vi "Correlation_coefficient.vi"(0 "U":dbl[](array[numeric]) format="%.2f", 1 "W":dbl[](array[numeric]) format="%.2f") -> (17 "Correlation coefficient":dbl format="%.2f")   [LabVIEW 2010]
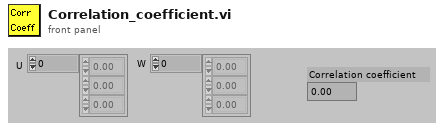
[diagram p1: front panel]
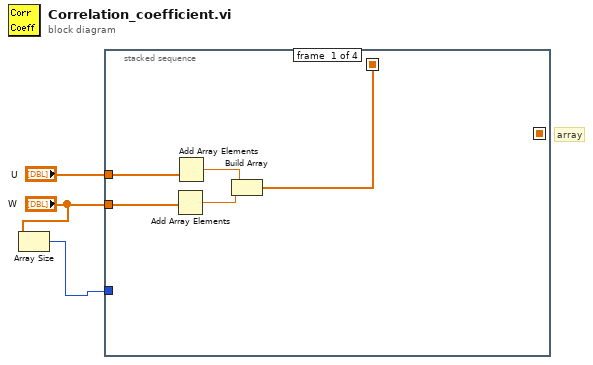
[diagram p0: block diagram]
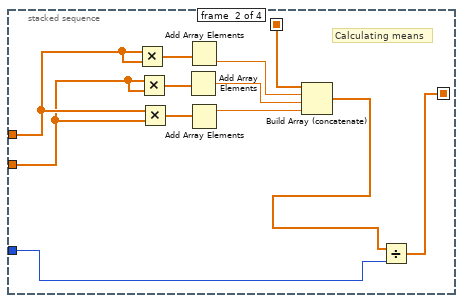
[diagram p2: hidden frame]
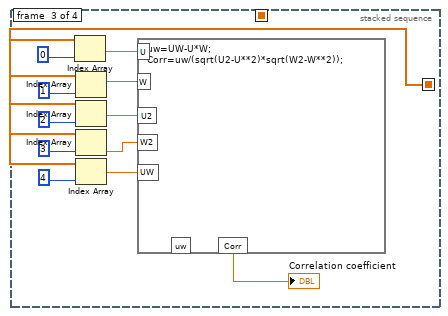
[diagram p3: hidden frame]
diagram:
  # "array"
  n1 = Array Size(array="W") -> (size(s)=w3:i32)
  n2 = stacked-sequence {
    seq-local: [_ w20 _ _] -> [_ _ w22 _]
    seq-local: [w4 _ _ _] -> [_ w16 _ _]
    tunnel: "U" -> [w8 w13 _ _]
    tunnel: w3 -> [_ w15 _ _]
    tunnel: "W" -> [w7 w12 _ _]
    frame #0 {
      n3 = Add Array Elements(numeric array=w7) -> (sum=w5:dbl)
      n4 = Add Array Elements(numeric array=w8) -> (sum=w6:dbl)
      n5 = Build Array(w6, w5) -> (w4:dbl[])
    }
    frame #1 {
      # "Calculating means"
      n6 = Multiply(x=w13, y=w13) -> (x*y=w9:dbl[])
      n7 = Multiply(x=w12, y=w12) -> (x*y=w10:dbl[])
      n8 = Multiply(x=w13, y=w12) -> (x*y=w11:dbl[])
      n9 = Add Array Elements(numeric array=w10) -> (sum=w19:dbl)
      n10 = Add Array Elements(numeric array=w9) -> (sum=w17:dbl)
      n11 = Add Array Elements(numeric array=w11) -> (sum=w18:dbl)
      n12 = Build Array (concatenate)(w16, w17, w19, w18) -> (w14:dbl[])
      n13 = Divide(x=w14, y=w15) -> (x/y=w20:dbl[])
    }
    frame #2 {
      n14 = Index Array(array=w22, index=0) -> (element=w27:dbl)
      n15 = Index Array(array=w22, index=1) -> (element=w26:dbl)
      n16 = Index Array(array=w22, index=2) -> (element=w25:dbl)
      n17 = Index Array(array=w22, index=3) -> (element=w24:dbl)
      n18 = Index Array(array=w22, index=4) -> (element=w23:dbl)
      n19 = formula code="uw=UW-U*W;\nCorr=uw/(sqrt(U2-U**2)*sqrt(W2-W**2));"("W"=w26, "W2"=w24, "U"=w27, "U2"=w25, "UW"=w23) -> ("Corr"=→"Correlation coefficient":dbl)  [unwired: 1 out]
    }
    frame #3 {
    }
  }
